vi "CIMAQ_Cast_Binary_RGB.vi"(8 "error in (no error)":errorcluster, 10 "Dest (optional)":T1=refnum, 11 "Source":T1) -> (0 "error out":errorcluster, 3 "Result":T1)   [LabVIEW 2017]
uses:
  <vilib>/vision/Image Controls.llb/IMAQ Image.ctl
  <vilib>/vision/NI_Vision_Development_Module.lvlib
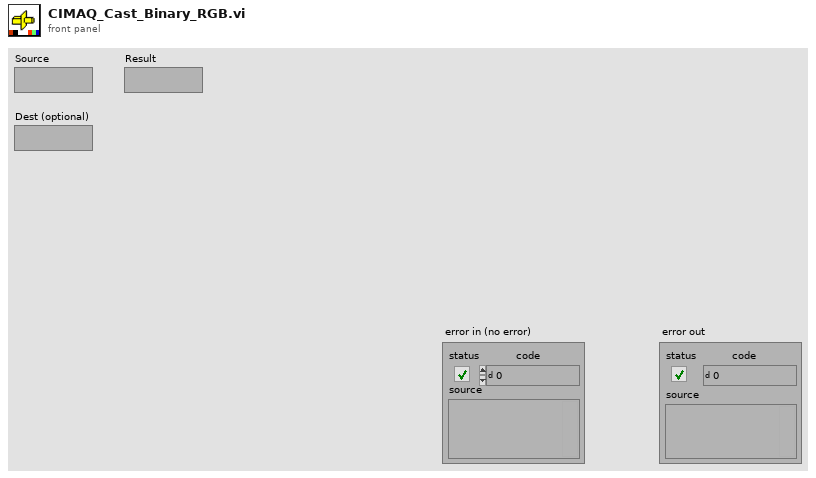
[diagram p1: front panel]
types:
  T1 = typedef "IMAQ Image.ctl" = refnum<image>
  T2 = enum32{"Gray", "Binary", "Gradient", "Rainbow", "Temperature"}
  T3 = typedef "Image Type" = u32
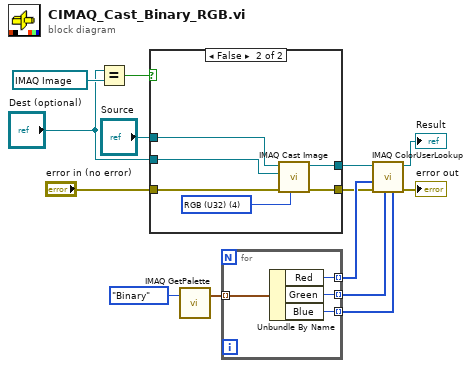
[diagram p0: block diagram]
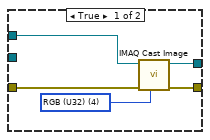
[diagram p2: hidden frame]
diagram:
  n1 = Equal?(x="Dest (optional)", y=T1 refnum ("Image Dst Out")) -> (x = y?=w5:bool)
  n2 = case shown="False" w5 {
    tunnel: [w18 w24] -> w14
    tunnel: "Source" -> [w17 w23]
    tunnel: "Dest (optional)" -> [_ w22]
    tunnel: "error in (no error)" -> [w16 w21]
    tunnel: [w15 w20] -> w2
    frame True {
      w19 = T3 4 items=["Grayscale (U8)", "Grayscale (I16)", "Grayscale (SGL)", "Complex (CSG)", "RGB (U32)", "HSL (U32)", "RGB (U64)", "Grayscale (U16)"] ("Image Type")
      n3 = call "IMAQ Cast Image"("Image Type"=w19, "error in (no error)"=w16, "Image Src"=w17) -> ("error out"=w15:errorcluster, "Image Dst Out"=w18:T1)  [unwired: 7 in]
    }
    frame False {
      w25 = T3 4 items=["Grayscale (U8)", "Grayscale (I16)", "Grayscale (SGL)", "Complex (CSG)", "RGB (U32)", "HSL (U32)", "RGB (U64)", "Grayscale (U16)"] ("Image Type")
      n4 = call "IMAQ Cast Image"("Image Type"=w25, "error in (no error)"=w21, "Image Dst"=w22, "Image Src"=w23) -> ("error out"=w20:errorcluster, "Image Dst Out"=w24:T1)  [unwired: 6 in]
    }
  }
  n5 = call "IMAQ GetPalette"("Palette Number (gray)"=T2."Binary") -> ("Color Palette"=w9:cluster{"Red":u8, "Green":u8, "Blue":u8}[])  [unwired: 4 in, 1 out]
  n6 = for {
    tunnel: w9 -> [w29] mode=indexing
    tunnel: [w28] -> w12 mode=indexing
    tunnel: [w27] -> w11 mode=indexing
    tunnel: [w26] -> w10 mode=indexing
    n7 = Unbundle By Name(w29) -> ("Red"=w26:u8, "Green"=w27:u8, "Blue"=w28:u8)
  }
  n8 = call "IMAQ ColorUserLookup"("Blue or Luma or Val or Inten Lookup Table"=w12, "Green or Sat Lookup Table"=w11, "error in (no error)"=w2, "Red or Hue Lookup Table"=w10, "Image Src"=w14) -> ("error out"=→"error out":errorcluster, "Image Dst Out"=→"Result":T1)  [unwired: 5 in]
